vi "Add Chassis.vi"(7 "Overwrite Existing?":bool=TRUE, 8 "error in (no error)":errorcluster, 9 "Settings":T2, 10 "Base Node Path":string, 11 "SysDef Ref":T3) -> (0 "error out":errorcluster, 2 "Chassis Node Paths":T1, 3 "SysDef Ref Out":T3)   [LabVIEW 2019, in "Simple SysDef API.lvlib"]
uses:
  <userlib>/SimpleSysDef/Simple SysDef API.lvlib
  <userlib>/SimpleSysDef/_SubVIs/System Definition Reference.ctl
  NationalInstruments.VeriStand.SystemDefinitionAPI
  <userlib>/SimpleSysDef/_SubVIs/Add Chassis_Settings.ctl
  <userlib>/SimpleSysDef/_SubVIs/Chassis Node Paths.ctl
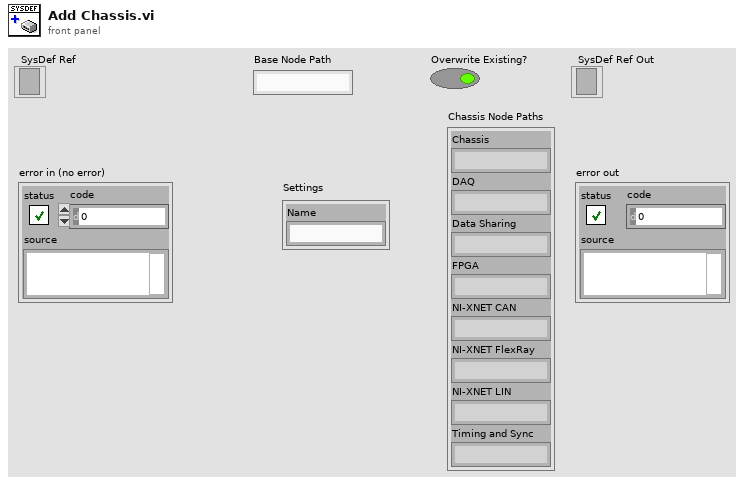
[diagram p1: front panel]
types:
  T1 = typedef "Simple SysDef API.lvlib/Chassis Node Paths.ctl" = cluster{"Chassis":string, "DAQ":string, "Data Sharing":string, "FPGA":string, "NI-XNET CAN":string, "NI-XNET FlexRay":string, "NI-XNET LIN":string, "Timing and Sync":string}
  T2 = typedef "Simple SysDef API.lvlib/Add Chassis_Settings.ctl" = cluster{"Name":string}
  T3 = typedef "Simple SysDef API.lvlib/System Definition Reference.ctl" = refnum<k24>
  T4 = cluster{"[0]":string, "[1]":string, "[2]":string, "[3]":string, "[4]":string, "[5]":string, "[6]":string, "[7]":string}
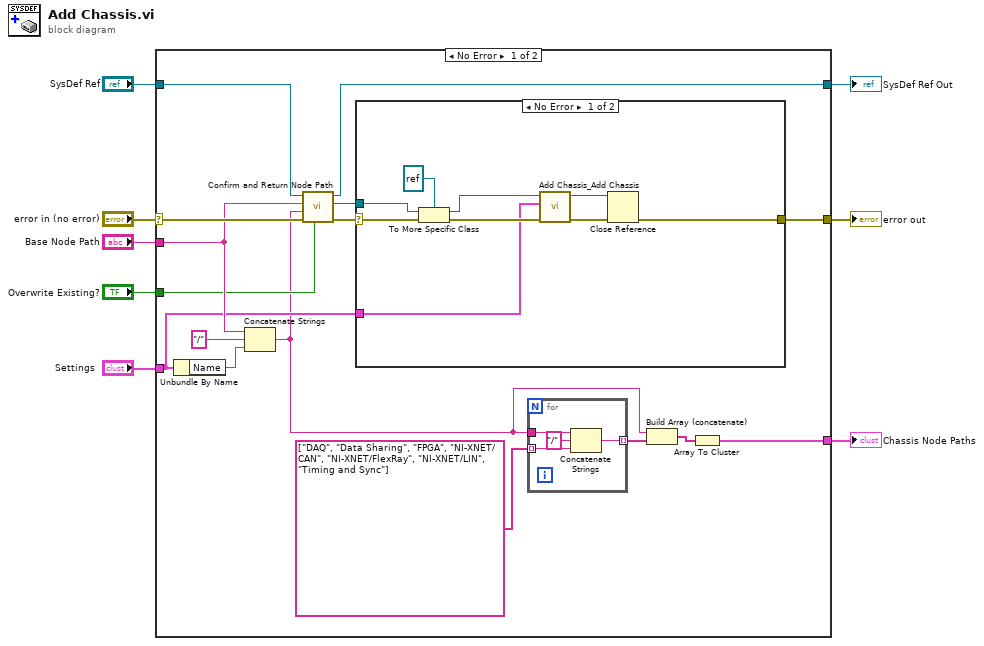
[diagram p0: block diagram]
diagram:
  n1 = case shown="No Error" "error in (no error)" {
    selector: "error in (no error)" -> [w24 w40]
    tunnel: [w19 w40] -> w7
    tunnel: "SysDef Ref" -> [w23 w39]
    tunnel: [w22 w39] -> w5
    tunnel: "Base Node Path" -> [w16 _]
    tunnel: "Overwrite Existing?" -> [w15 _]
    tunnel: "Settings" -> [w11 _]
    tunnel: [w12 _] -> w1
    frame No Error {
      n2 = Unbundle By Name(w11) -> ("Name"=w20:string)
      n3 = Concatenate Strings(w16, "/" ("string"), w20) -> (w9:string)
      n4 = call <userlib>:"Confirm and Return Node Path.vi"("Overwrite Existing?"=w15, "error in (no error)"=w24, "New Node Path"=w9, "Base Node Path"=w16, "SysDef Ref"=w23) -> ("error out"=w17:errorcluster, "Node Ref"=w18:refnum<k24>, "SysDef Ref Out"=w22:T3)  [unwired: 4 in]
      n5 = case shown="No Error" w17 {
        selector: w17 -> [w36 w38]
        tunnel: [w29 w38] -> w19
        tunnel: w18 -> [w37 _]
        tunnel: w11 -> [w32 _]
        frame No Error {
          n6 = To More Specific Class(target class=refnum<k24> refnum ("Node Ref"), reference=w37, error in=w36) -> (specific class reference=w34:refnum<k24>, error out=w33:errorcluster)
          n7 = call <userlib>:"Add Chassis_Add Chassis.vi"("error in (no error)"=w33, "Settings"=w32, "Hardware Ref"=w34) -> ("error out"=w30:errorcluster, "Hardware Ref Out"=w31:refnum<k24>)  [unwired: 7 in]
          n8 = Close Reference(reference=w31, error in (no error)=w30) -> (error out=w29:errorcluster)
        }
        frame Error {
        }
      }
      n9 = for {
        tunnel: w9 -> [w28]
        tunnel: string[] ["DAQ", "Data Sharing", "FPGA", "NI-XNET/CAN", "NI-XNET/FlexRay", "NI-XNET/LIN", "Timing and Sync"] -> [w26] mode=indexing
        tunnel: [w25] -> w13 mode=indexing
        n10 = Concatenate Strings(w28, "/" ("string"), w26) -> (w25:string)
      }
      n11 = Build Array (concatenate)(w9, w13) -> (w10:string[])
      n12 = Array To Cluster(array=w10) -> (cluster=w12:T4)
    }
    frame Error {
    }
  }
  "SysDef Ref Out" <- w5
  "error out" <- w7
  "Chassis Node Paths" <- w1
